vi "toBooleanSpectrum.vi"(2 "value_in":u8[](array[numeric]), 3 "dim_y":i32, 4 "dim_x":i32) -> (0 "setpoint":bool[](array[boolean]), 1 "value_out":bool[](array[boolean]))   [LabVIEW 2014, in "tango.lvlib"]
uses:
  tango.lvlib
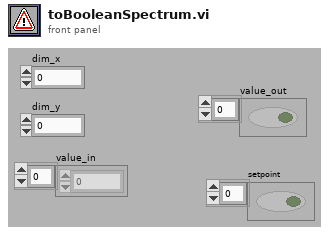
[diagram p1: front panel]
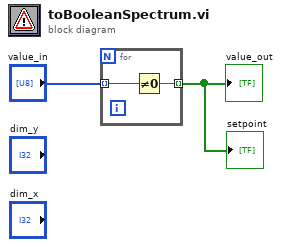
[diagram p0: block diagram]
diagram:
  n1 = for {
    tunnel: "value_in" -> [w4] mode=indexing
    tunnel: [w3] -> w1 mode=indexing
    n2 = Not Equal To 0?(x=w4) -> (x != 0?=w3:bool)
  }
  "value_out" <- w1
  "setpoint" <- w1
